vi "Configure Range.vi"   [LabVIEW 2021, in "Yokogawa WT1800 Series.lvlib"]
doc: "Configures the range features."
uses:
  <instrlib>/Yokogawa WT1800 Series/Yokogawa WT1800 Series.lvlib
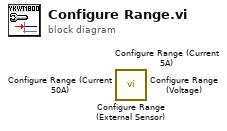
[diagram p0: block diagram]
diagram:
  n1 = call <instrlib>:"Configure Range (External Sensor).vi"() -> ()  [unwired: 14 in, 2 out]
  n2 = call <instrlib>:"Configure Range (Current 5A).vi"() -> ()  [unwired: 14 in, 2 out]
  n3 = call <instrlib>:"Configure Range (Current 50A).vi"() -> ()  [unwired: 14 in, 2 out]
  n4 = call <instrlib>:"Configure Range (Voltage).vi"() -> ()  [unwired: 14 in, 2 out]
